vi "Do.vi"(8 "error in (no error)":errorcluster, 9 "CommandQueueIn":refnum<queue>, 10 "DataNotifierIn":refnum<notifier>, 11 "CommandCopy in":refnum<class "CSVExport.lvclass">) -> (0 "error out":errorcluster, 1 "ExitFlag":bool, 2 "DataNotifierOut":refnum<notifier>, 3 "CommandCopy out":refnum<class "CSVExport.lvclass">)   [LabVIEW 2013, in "CSVExport.lvclass"]
uses:
  CSVExport.lvclass
  SystemData.lvclass/SystemData.lvclass
  RootCommand.lvclass/RootCommand.lvclass
  SystemData.lvclass/SystemData.lvclass/SystemData.ctl
  <vilib>/Utility/file.llb/Write To Spreadsheet File (DBL).vi
  Generator.lvclass/Generator.lvclass
panel:
  # "notifier包裝SystemData物件的參考"
  # "命令物件序列參考"
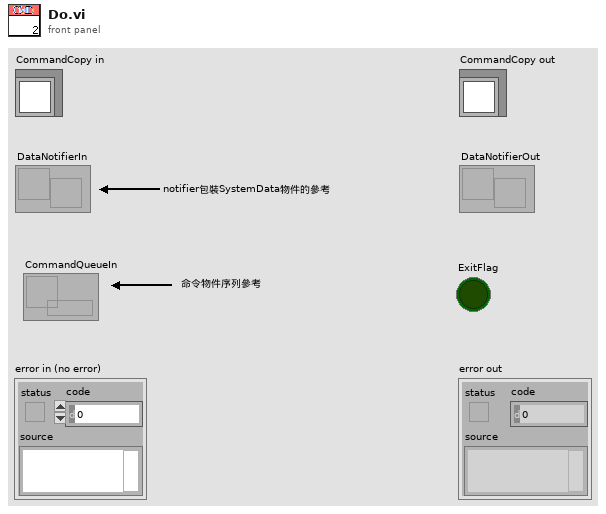
[diagram p1: front panel]
types:
  T1 = typedef "SystemData.lvclass/SystemDataTypeDefine.ctl" = cluster{"ThisVIParameter":cluster{"ThisVIPath":path, "ThisVIReference":refnum<vi>, "AllControlReference":refnum<vi>[]}, "GeneratorParameter":cluster{"Frequency":dbl, "Amplitude":dbl}, "WaveformBuffer":waveform(dbl), "SourceSelect":u16, "GeneratorClassArray":refnum<class "Generator.lvclass">[]}
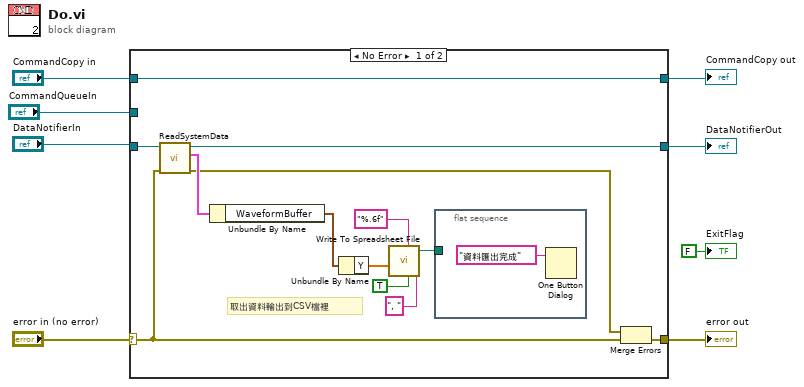
[diagram p0: block diagram]
diagram:
  n1 = case shown="No Error" "error in (no error)" {
    selector: "error in (no error)" -> [w17 w25]
    tunnel: [w18 w25] -> w4
    tunnel: [w21 w24] -> w3
    tunnel: "CommandCopy in" -> [w21 w24]
    tunnel: "DataNotifierIn" -> [w20 w23]
    tunnel: [w11 w23] -> w2
    tunnel: "CommandQueueIn" -> [_ _]
    frame No Error {
      # "取出資料輸出到CSV檔裡"
      n2 = call "ReadSystemData.vi"("error in (no error)"=w17, "DataNotifierIn"=w20) -> ("error out"=w10:errorcluster, "SystemData"=w19:T1, "DataNotifierIn"=w11:refnum<notifier>)  [unwired: 7 in]
      n3 = Unbundle By Name(w19) -> ("WaveformBuffer"=w16:waveform(dbl))
      n4 = Unbundle By Name(w16) -> ("Y"=w15:dbl[])
      n5 = call-poly <vilib>:"Write To Spreadsheet File.vi"("delimiter (\\t)"=", " ("delimiter (\\t)"), "transpose? (no:F)"=TRUE, "format (%.3f)"="%.6f", "1D data"=w15) -> ("new file path (Not A Path if cancelled)"=w9:path)  [unwired: 4 in]
      n6 = flat-sequence {
        tunnel: w9 -> [_]
        frame #0 {
          n7 = One Button Dialog(message="資料匯出完成") -> ()  [unwired: 1 in, 1 out]
        }
      }
      n8 = Merge Errors(w10, w17) -> (w18:errorcluster)
    }
    frame Error {
    }
  }
  "error out" <- w4
  "CommandCopy out" <- w3
  "DataNotifierOut" <- w2
  "ExitFlag" <- FALSE ("ExitFlag")
